vi "Configure Average.vi"(7 "Average On":bool, 8 "error in (no error)":errorcluster, 10 "Number of Averages":i32, 11 "VNA-CMT S2 S4 in":refnum<class "VNA-CMT S2 S4.lvclass">) -> (0 "error out":errorcluster, 3 "VNA-CMT S2 S4 out":refnum<class "VNA-CMT S2 S4.lvclass">)   [LabVIEW 2020, in "VNA-CMT S2 S4.lvclass"]
doc: "Configures the average to use for the sweep"
uses:
  VNA-CMT S2 S4.lvclass
  C:/Sandbox/RF Bench/Source Code/WiSpry Test Framework/Instruments/Instrument.lvclass
  Instrument.lvclass/Instrument.ctl
  Instrument.lvclass
  <instrlib>/CMT S2 and S4 VNA/CMT S2 and S4 VNA.lvlib
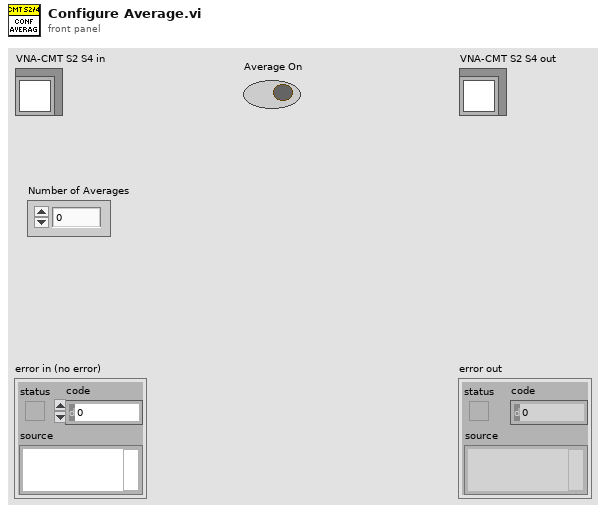
[diagram p1: front panel]
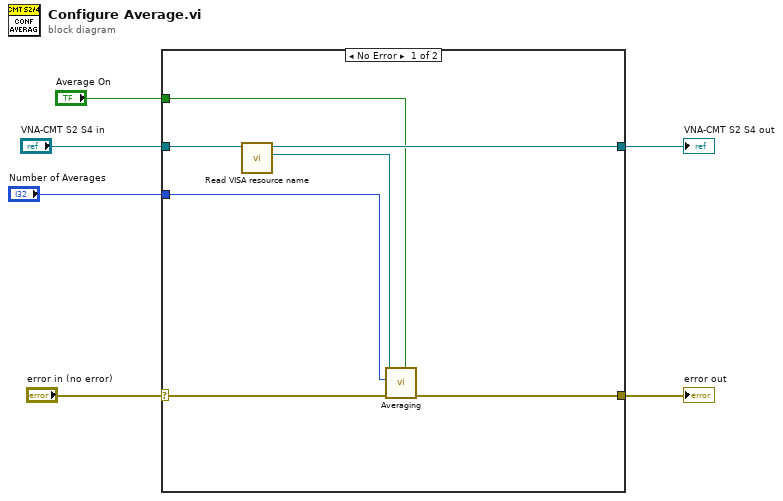
[diagram p0: block diagram]
diagram:
  n1 = case shown="No Error" "error in (no error)" {
    selector: "error in (no error)" -> [w8 w14]
    tunnel: "VNA-CMT S2 S4 in" -> [w13 w15]
    tunnel: [w12 w15] -> w4
    tunnel: [w7 w14] -> w3
    tunnel: "Average On" -> [w11 _]
    tunnel: "Number of Averages" -> [w10 _]
    frame No Error {
      n2 = call "Read VISA resource name.vi"("Instrument in"=w13) -> ("VISA resource name"=w9:refnum<visa-resource-name>, "Instrument out"=w12:refnum<class "VNA-CMT S2 S4.lvclass">)  [unwired: 9 in]
      n3 = call <instrlib>:"Averaging.vi"("Averaging State (F: Off)"=w11, "error in (no error)"=w8, "Factor (10)"=w10, "VISA resource name"=w9) -> ("error out"=w7:errorcluster)  [unwired: 6 in, 1 out]
    }
    frame Error {
    }
  }
  "error out" <- w3
  "VNA-CMT S2 S4 out" <- w4
